vi "testsubinitialize.vi"(4 "Exposure Time (secs)":sgl format="%.2f", 5 "Trigger":u32(ring) items=["Internal", "External"]) -> (0 "Camera outputs":T3, 1 "Camera status":T1, 2 "Camera inputs":T2)   [LabVIEW 2017]
uses:
  atmcd32d.dll
panel:
  out "to shutdown":bool
  out "DRV_SUCCESS":i32
  out "to start acquisition":bool
  out "to get acquired data":bool
  out "Set Image":u32
  out "Set Gate Mode":u32
  out "Detector Y Pixels":i32
  out "Get Detector":u32
  out "Set Exposure Time":u32
  out "Set Trigger Mode":u32
  out "Set Readout Mode":u32
  out "Set Acquisition Mode":u32
  out "Check Timings":u32
  out "Detector X Pixels":i32
  out "Calculated Exposure Value":sgl format="%.5f"
  out "Initialize":u32
  # "Status"
  # "Return values"
  # "USB iStarIMAG32at.VI"
  # "Acquisition Mode: Single Scan\nReadout Mode: Full Resolution Image"
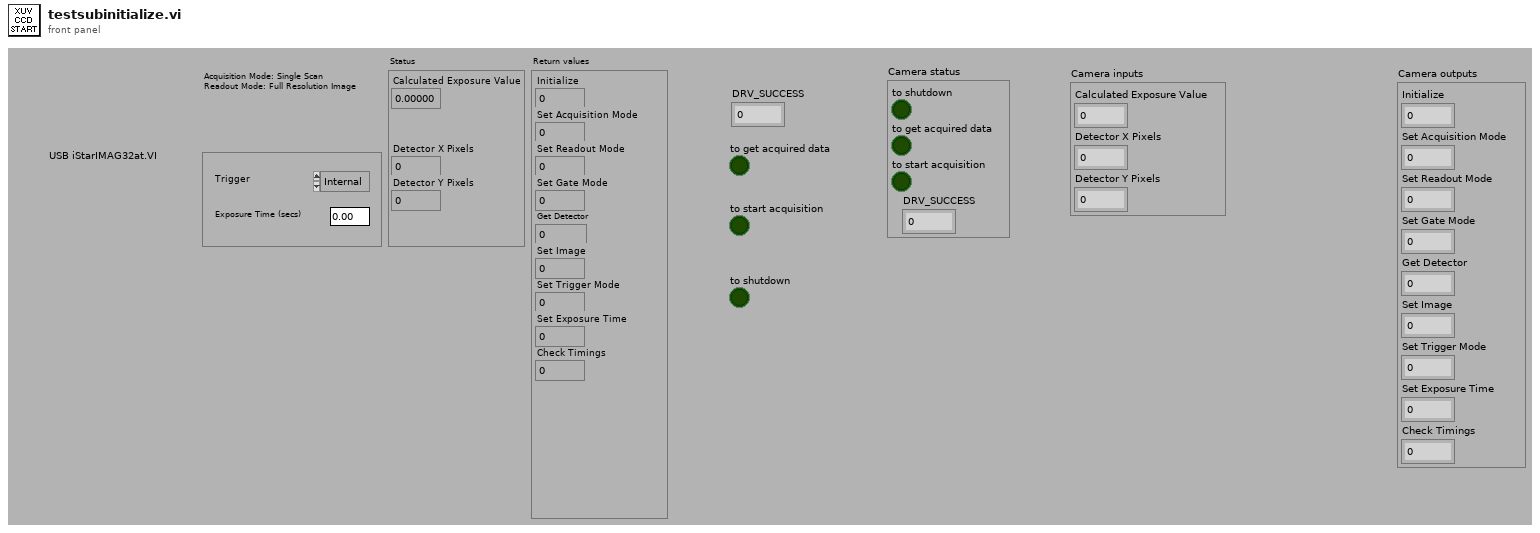
[diagram p1: front panel]
types:
  T1 = cluster{"to shutdown":bool, "to get acquired data":bool, "to start acquisition":bool, "DRV_SUCCESS":i32}
  T2 = cluster{"Calculated Exposure Value":sgl, "Detector X Pixels":i32, "Detector Y Pixels":i32}
  T3 = cluster{"Initialize":u32, "Set Acquisition Mode":u32, "Set Readout Mode":u32, "Set Gate Mode":u32, "Get Detector":u32, "Set Image":u32, "Set Trigger Mode":u32, "Set Exposure Time":u32, "Check Timings":u32}
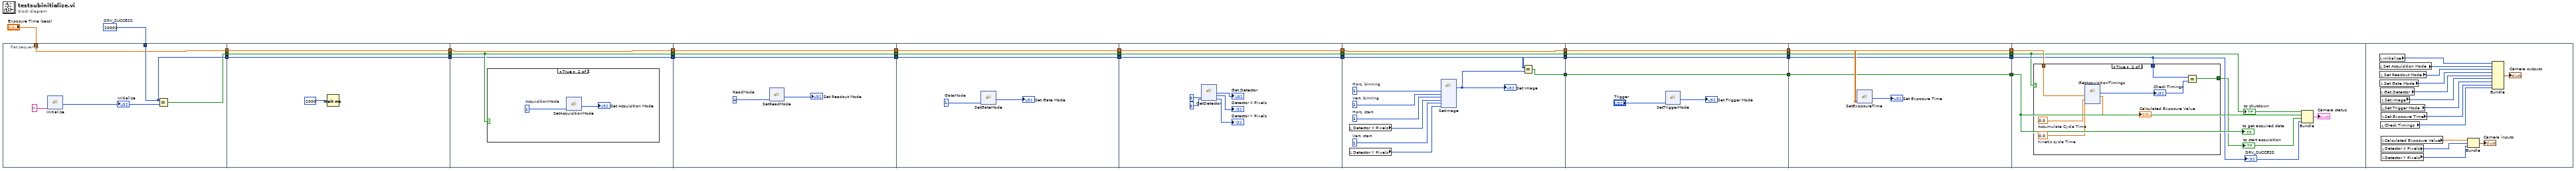
[diagram p0: block diagram]
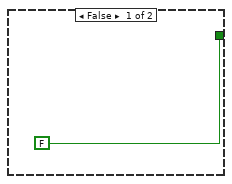
[diagram p3: hidden frame]
diagram:
  w31 = 20002  # DRV_SUCCESS
  n1 = flat-sequence {
    tunnel: "Exposure Time (secs)" -> [w33]
    tunnel: [w33] -> w30
    tunnel: w31 -> [w36]
    tunnel: [w36] -> w29
    tunnel: [w35] -> w28
    tunnel: w30 -> [w40]
    tunnel: [w40] -> w27
    tunnel: w29 -> [w39]
    tunnel: [w39] -> w26
    tunnel: w28 -> [w38]
    tunnel: [w38] -> w25
    tunnel: w27 -> [w43]
    tunnel: [w43] -> w24
    tunnel: w26 -> [w42]
    tunnel: [w42] -> w23
    tunnel: w25 -> [w44]
    tunnel: [w44] -> w22
    tunnel: w24 -> [w49]
    tunnel: [w49] -> w21
    tunnel: w23 -> [w48]
    tunnel: [w48] -> w20
    tunnel: w22 -> [w47]
    tunnel: [w47] -> w19
    tunnel: w21 -> [w54]
    tunnel: [w54] -> w18
    tunnel: w20 -> [w53]
    tunnel: [w53] -> w17
    tunnel: w19 -> [w52]
    tunnel: [w52] -> w16
    tunnel: w18 -> [w59]
    tunnel: [w59] -> w15
    tunnel: w17 -> [w58]
    tunnel: [w58] -> w14
    tunnel: w16 -> [w57]
    tunnel: [w57] -> w13
    tunnel: w15 -> [w66]
    tunnel: [w66] -> w12
    tunnel: w14 -> [w69]
    tunnel: [w69] -> w11
    tunnel: w13 -> [w65]
    tunnel: [w65] -> w10
    tunnel: [w67] -> w9
    tunnel: w12 -> [w79]
    tunnel: [w79] -> w8
    tunnel: w11 -> [w78]
    tunnel: [w78] -> w7
    tunnel: w10 -> [w77]
    tunnel: [w77] -> w6
    tunnel: w9 -> [w76]
    tunnel: [w76] -> w5
    tunnel: w8 -> [w86]
    tunnel: [w86] -> w4
    tunnel: w7 -> [w84]
    tunnel: [w84] -> w3
    tunnel: w6 -> [w83]
    tunnel: [w83] -> w2
    tunnel: w5 -> [w82]
    tunnel: [w82] -> w1
    tunnel: w4 -> [w92]
    tunnel: w3 -> [w91]
    tunnel: w2 -> [w89]
    tunnel: w1 -> [w88]
    frame #0 {
      n2 = dll-call lib="atmcd32d.dll" fn="Initialize" label="Call Library Function Initialize"("") -> (w37:u32)  [unwired: 4 in, 2 out]
      "Initialize" <- w37
      n3 = Equal?(x=w36, y=w37) -> (x = y?=w35:bool)
    }
    frame #1 {
      n4 = Wait (ms)(milliseconds to wait=u32 2000) -> ()  [unwired: 1 out]
    }
    frame #2 {
      n5 = case shown="True" w44 {
        frame False {
        }
        frame True {
          w46 = u16 1  # AcquisitionMode
          n6 = dll-call lib="atmcd32d.dll" fn="SetAcquisitionMode" label="Call Library Function SetAcquisitionMode"(w46) -> (→"Set Acquisition Mode":u32)  [unwired: 4 in, 2 out]
        }
      }
    }
    frame #3 {
      w51 = u16 4  # ReadMode
      n7 = dll-call lib="atmcd32d.dll" fn="SetReadMode" label="Call Library Function SetReadMode"(w51) -> (→"Set Readout Mode":u32)  [unwired: 4 in, 2 out]
    }
    frame #4 {
      w56 = u16 1  # GateMode
      n8 = dll-call lib="atmcd32d.dll" fn="SetGateMode" label="Call Library Function SetGateMode"(w56) -> (→"Set Gate Mode":u32)  [unwired: 4 in, 2 out]
    }
    frame #5 {
      n9 = dll-call lib="atmcd32d.dll" fn="GetDetector" label="Call Library FunctionGetDetector"(i16 0, i16 0) -> (→"Get Detector":u32, →"Detector X Pixels":i32, →"Detector Y Pixels":i32)  [unwired: 3 in, 2 out]
    }
    frame #6 {
      w72 = u16 1  # Vert. start
      w73 = u16 1  # Horz. start
      w74 = u16 1  # Vert. binning
      w75 = u16 1  # Horz. binning
      n10 = local read "Detector X Pixels"() -> (w71:i32)
      n11 = local read "Detector Y Pixels"() -> (w70:i32)
      n12 = dll-call lib="atmcd32d.dll" fn="SetImage" label="Call Library Function SetImage"(w75, w74, w73, w71, w72, w70) -> (w68:u32)  [unwired: 9 in, 2 out]
      "Set Image" <- w68
      n13 = Equal?(x=w69, y=w68) -> (x = y?=w67:bool)
    }
    frame #7 {
      n14 = dll-call lib="atmcd32d.dll" fn="SetTriggerMode" label="Call Library Function SetTrigger Mode"("Trigger") -> (→"Set Trigger Mode":u32)  [unwired: 4 in, 2 out]
    }
    frame #8 {
      n15 = dll-call lib="atmcd32d.dll" fn="SetExposureTime" label="Call Library FunctionSet Exposure Time"(w86) -> (→"Set Exposure Time":u32)  [unwired: 4 in, 2 out]
    }
    frame #9 {
      n16 = case shown="True" w89 {
        tunnel: w92 -> [_ w97]
        tunnel: w91 -> [_ w94]
        tunnel: [FALSE w96] -> w87
        frame False {
        }
        frame True {
          w99 = sgl 0.0  # Accumulate Cycle Time
          w100 = sgl 0.0  # Kinetic cycle Time
          n17 = dll-call lib="atmcd32d.dll" fn="GetAcquisitionTimings" label="Call Library Function Check Timings"(w97, w99, w100) -> (w95:u32, →"Calculated Exposure Value":sgl)  [unwired: 5 in, 2 out]
          "Check Timings" <- w95
          n18 = Equal?(x=w94, y=w95) -> (x = y?=w96:bool)
        }
      }
      "to start acquisition" <- w87
      n19 = Bundle(w89, w88, w87, "DRV_SUCCESS"=w91) -> (→"Camera status":cluster{bool, bool, bool, "DRV_SUCCESS":i32})  [unwired: 1 in]
      "to get acquired data" <- w88
      "DRV_SUCCESS" <- w91
      "to shutdown" <- w89
    }
    frame #10 {
      n20 = local read "Initialize"() -> (w114:u32)
      n21 = local read "Set Acquisition Mode"() -> (w113:u32)
      n22 = local read "Set Readout Mode"() -> (w112:u32)
      n23 = local read "Set Gate Mode"() -> (w111:u32)
      n24 = local read "Get Detector"() -> (w110:u32)
      n25 = local read "Set Image"() -> (w109:u32)
      n26 = local read "Check Timings"() -> (w106:u32)
      n27 = local read "Set Trigger Mode"() -> (w108:u32)
      n28 = local read "Set Exposure Time"() -> (w107:u32)
      n29 = local read "Calculated Exposure Value"() -> (w104:sgl)
      n30 = local read "Detector X Pixels"() -> (w103:i32)
      n31 = local read "Detector Y Pixels"() -> (w102:i32)
      n32 = Bundle("Calculated Exposure Value"=w104, "Detector X Pixels"=w103, "Detector Y Pixels"=w102) -> (→"Camera inputs":T2)  [unwired: 1 in]
      n33 = Bundle("Initialize"=w114, "Set Acquisition Mode"=w113, "Set Readout Mode"=w112, "Set Gate Mode"=w111, "Get Detector"=w110, "Set Image"=w109, "Set Trigger Mode"=w108, "Set Exposure Time"=w107, "Check Timings"=w106) -> (→"Camera outputs":T3)  [unwired: 1 in]
    }
  }
